vi "Select sys configs.vi"(8 "error in (no error)":errorcluster) -> (0 "error out":errorcluster, 1 "SysdefSettings":T1, 3 "paths":path[](array[path]), 4 "Target IP Address":string, 5 "Tolerence (%)":dbl=2.0, 6 "Log file":path, 7 "Converge target (Hz)":dbl=50.0)   [LabVIEW 2011]
uses:
  Sysdef Settings.ctl
panel:
  in  "DAQ_ConvClock":bool
  in  "DAQ_SampCompl":bool
  in  "Target IP":string
  in  "Result log file":path
  in  "Pass/fail within":dbl=3.0
  in  "Converge to nearest":dbl=50.0
  in  "Cancel":bool
  in  "OK":bool
  in  "Path":path
  # "Select a directory of system configurations (*.nivssdf) you wish to benchmark."
  # "Hz"
  # "% tolerance"
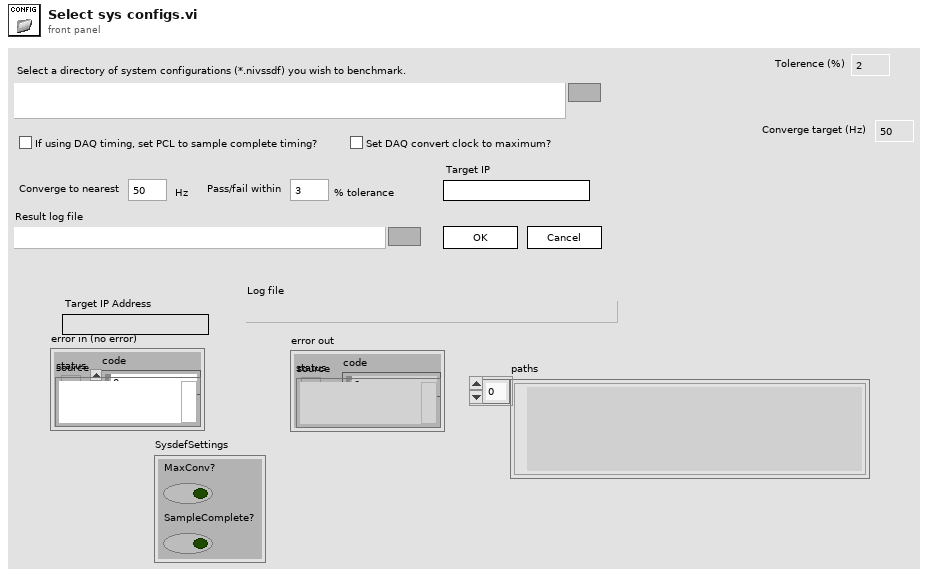
[diagram p1: front panel]
types:
  T1 = typedef "Sysdef Settings.ctl" = cluster{"MaxConv?":bool, "SampleComplete?":bool}
  T2 = enum8{"Enabled", "Disabled", "Disabled and Grayed Out"}
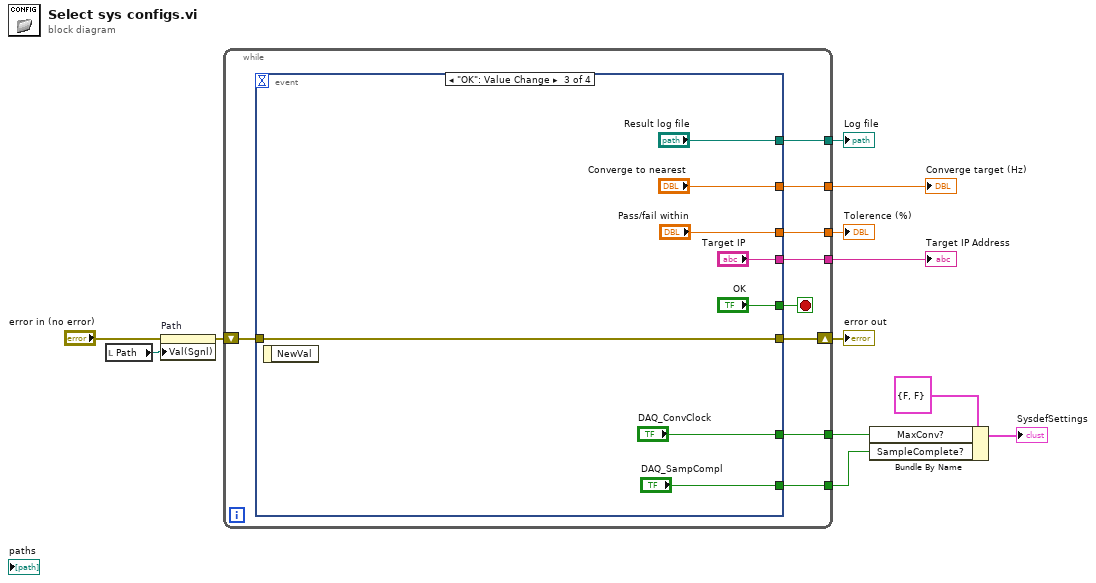
[diagram p0: block diagram]
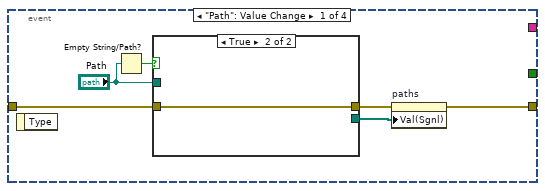
[diagram p2: hidden frame]
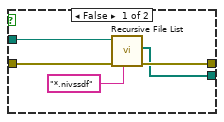
[diagram p3: hidden frame]
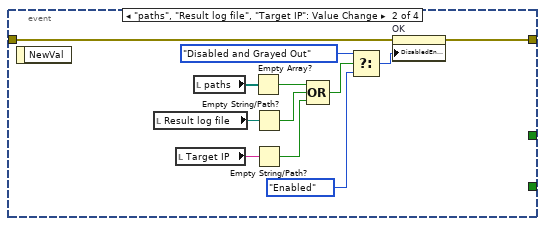
[diagram p4: hidden frame]
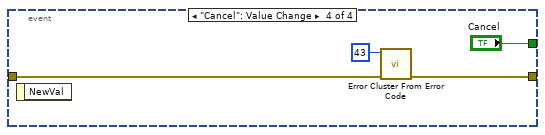
[diagram p5: hidden frame]
diagram:
  n1 = local read "Path"() -> (w6:path)
  n2 = property on="Path" class="Path"(error in="error in (no error)", "Val(Sgnl)"=w6) -> (error out=w11:errorcluster)  [unwired: 1 in, 1 out]
  n3 = while {
    shift-right: [w20] -> w12
    shift-left: w11 -> [w21]
    tunnel: [w18] -> w10
    tunnel: [w17] -> w9
    tunnel: [w16] -> w8
    tunnel: [w15] -> w5
    tunnel: [w14] -> w1
    tunnel: [w13] -> w2
    stop <- w19 stop-if-true
    n4 = event shown="[2] \"OK\": Value Change" {
      selector: _ -> [_ _ _ _]
      dyn-events: _ -> [_ _ _ _]
      timeout: _ -> [_ _ _ _]
      tunnel: w21 -> [w27 w45 w52 w55]
      tunnel: [w25 w44 w52 w56] -> w20
      tunnel: [_ _ "OK" "Cancel"] -> w19
      tunnel: [_ _ "Converge to nearest" _] -> w18
      tunnel: [_ _ "Pass/fail within" _] -> w17
      tunnel: [_ _ "Result log file" _] -> w16
      tunnel: [_ _ "Target IP" _] -> w15
      tunnel: [_ _ "DAQ_SampCompl" _] -> w14
      tunnel: [_ _ "DAQ_ConvClock" _] -> w13
      event "Path": Value Change {
        n5 = event-data() -> ()  [unwired: 1 in, 1 out]
        n6 = Empty String/Path?(string/path="Path") -> (empty?=w22:bool)
        n7 = case shown="True" w22 {
          tunnel: "Path" -> [w32 _]
          tunnel: w27 -> [w31 w33]
          tunnel: [w29 w33] -> w26
          tunnel: [w28 _] -> w24
          frame False {
            n8 = call <vilib>:"Recursive File List.vi"("pattern"="*.nivssdf", "error in (no error)"=w31, "Folder Path"=w32) -> ("error out"=w29:errorcluster, "All Files in Dir"=w28:path[])  [unwired: 4 in, 3 out]
          }
          frame True {
          }
        }
        n9 = property on="paths" class="Arr (strict)"(error in=w26, "Val(Sgnl)"=w24) -> (error out=w25:errorcluster)  [unwired: 1 in, 1 out]
      }
      event "paths", "Result log file", "Target IP": Value Change {
        n10 = event-data() -> ()  [unwired: 1 in, 1 out]
        n11 = local read "Result log file"() -> (w37:path)
        n12 = local read "Target IP"() -> (w35:string)
        n13 = local read "paths"() -> (w39:path[])
        n14 = Empty Array?(array=w39) -> (empty?=w43:bool)
        n15 = Empty String/Path?(string/path=w37) -> (empty?=w36:bool)
        n16 = Empty String/Path?(string/path=w35) -> (empty?=w34:bool)
        n17 = Compound Arithmetic op=OR(w43, w36, w34) -> (w38:bool)
        n18 = Select(t=T2."Disabled and Grayed Out" ("Disabled"), s=w38, f=T2."Enabled") -> (s? t:f=w41:T2)
        n19 = property on="OK" class="Bool"(error in=w45, "DisabledEnum"=w41) -> (error out=w44:errorcluster)  [unwired: 1 in, 1 out]
      }
      event "OK": Value Change {
        n20 = event-data() -> ()  [unwired: 1 in, 1 out]
      }
      event "Cancel": Value Change {
        n21 = event-data() -> ()  [unwired: 1 in, 1 out]
        n22 = call <vilib>:"Error Cluster From Error Code.vi"("error in (no error)"=w55, "error code (0)"=43) -> ("error out"=w56:errorcluster)  [unwired: 7 in]
      }
    }
  }
  "error out" <- w12
  "Tolerence (%)" <- w9
  "Converge target (Hz)" <- w10
  "Log file" <- w8
  "Target IP Address" <- w5
  n23 = Bundle By Name(cluster=T1 {"MaxConv?"=FALSE, "SampleComplete?"=FALSE} ("SysdefSettings"), "MaxConv?"=w2, "SampleComplete?"=w1) -> (→"SysdefSettings":T1)
